vi "GetPressure.vi"(8 "error in (no error)":errorcluster, 11 "SimGauge in":refnum<class "SimGauge.lvclass">) -> (0 "error out":errorcluster, 2 "Pressure (mbar)":dbl, 3 "SimGauge out":refnum<class "SimGauge.lvclass">)   [LabVIEW 2016, in "SimGauge.lvlib" / "SimGauge.lvclass"]
uses:
  SimGauge.lvclass
  SimGauge.lvclass/SimGauge.ctl
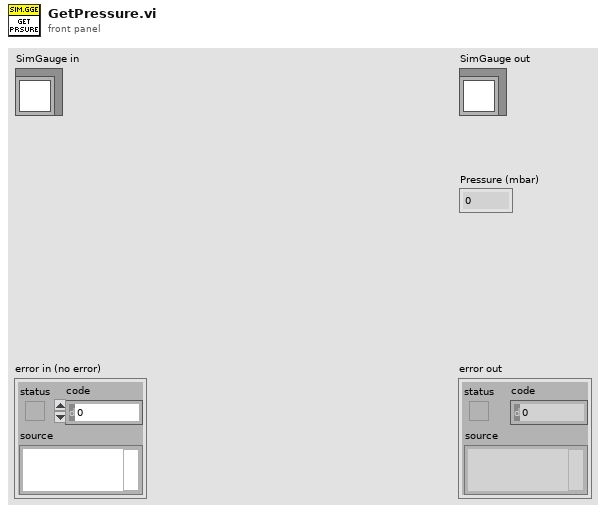
[diagram p1: front panel]
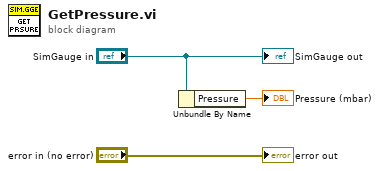
[diagram p0: block diagram]
diagram:
  n1 = Unbundle By Name("SimGauge in") -> ("Pressure"=→"Pressure (mbar)":dbl)
  "error out" <- "error in (no error)"
  "SimGauge out" <- "SimGauge in"
